vi "Encoder Angles.vi"(8 "calibration angle":dbl, 9 "low voltage":dbl, 10 "top voltage":dbl, 11 "AIDeviceRef Encoder":T1={"DevStatus"={"status"=FALSE, "code"=0, "source"=""}, "Controller"=enum."Controller 1", "Analog Channel"=enum."AI 1"}) -> (3 "encoder angle":dbl)   [LabVIEW 2014]
uses:
  <vilib>/Rock Robotics/WPI/AnalogChannel/WPI_AnalogChannelDevRef.ctl
  <vilib>/Rock Robotics/SystemInterfaces/Typedef/FPGA_TypedefAnalogModule.ctl
  <vilib>/Rock Robotics/SystemInterfaces/AI/FPGA_AIChannel.ctl
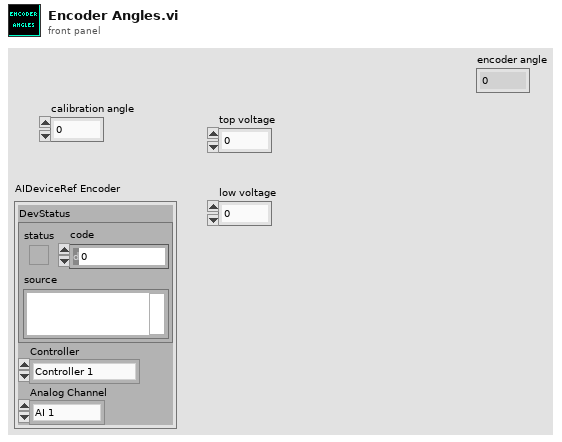
[diagram p1: front panel]
types:
  T1 = typedef "WPI_AnalogChannelDevRef.ctl" = cluster{"DevStatus":errorcluster, "Controller":T2, "Analog Channel":T3}
  T2 = typedef "FPGA_TypedefAnalogModule.ctl" = enum16{"Controller 1"}
  T3 = typedef "FPGA_AIChannel.ctl" = enum8{"AI 0", "AI 1", "AI 2", "AI 3", "AI MXP 0", "AI MXP 1", "AI MXP 2", "AI MXP 3", "Invalid"}
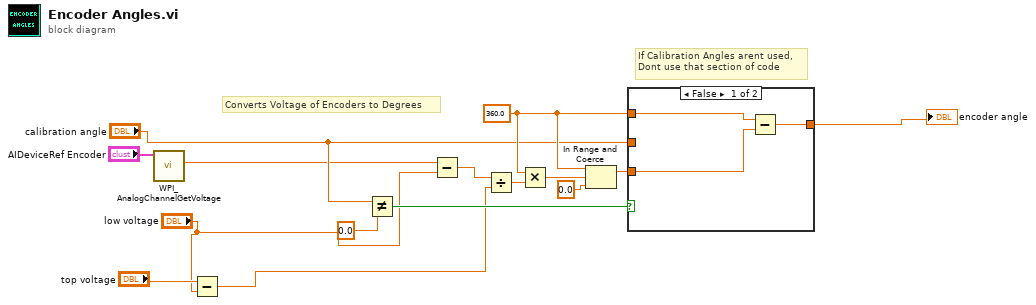
[diagram p0: block diagram]
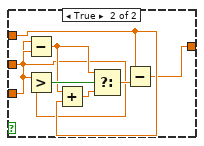
[diagram p2: hidden frame]
diagram:
  w11 = 360.0 ("y")
  # "Converts Voltage of Encoders to Degrees"
  # "If Calibration Angles arent used,\nDont use that section of code"
  n1 = call <vilib>:"WPI_AnalogChannelGetVoltage.vi"("AIDeviceRef"="AIDeviceRef Encoder") -> ("Voltage"=w2:dbl)  [unwired: 8 in, 2 out]
  n2 = Subtract(x="top voltage", y="low voltage") -> (x-y=w4:dbl)
  n3 = Not Equal?(x="calibration angle", y=0.0) -> (x != y?=w9:bool)
  n4 = Subtract(x=w2, y="low voltage") -> (x-y=w15:dbl)
  n5 = Divide(x=w15, y=w4) -> (x/y=w14:dbl)
  n6 = Multiply(x=w11, y=w14) -> (x*y=w13:dbl)
  n7 = In Range and Coerce(upper limit=w11, x=w13, lower limit=0.0) -> (coerced(x)=w10:dbl)  [unwired: 1 out]
  n8 = case shown="False" w9 {
    tunnel: w11 -> [w16 w22]
    tunnel: "calibration angle" -> [_ w21]
    tunnel: w10 -> [w17 w20]
    tunnel: [w18 w19] -> w1
    frame False {
      n9 = Subtract(x=w16, y=w17) -> (x-y=w18:dbl)
    }
    frame True {
      n10 = Subtract(x=w20, y=w21) -> (x-y=w25:dbl)
      n11 = Greater?(x=w20, y=w21) -> (0:w26:bool)
      n12 = Add(x=w25, y=w22) -> (x+y=w24:dbl)
      n13 = Select(t=w25, s=w26, f=w24) -> (s? t:f=w23:dbl)
      n14 = Subtract(x=w22, y=w23) -> (x-y=w19:dbl)
    }
  }
  "encoder angle" <- w1
